vi "Complex Dot Product (no conjugate).vi"(2 "Y Vector":cdb[](array[numeric]), 3 "X Vector":cdb[](array[numeric])) -> (0 "error":i32, 1 "X * Y":cdb)   [LabVIEW 2018, in "NI_AALBase.lvlib"]
doc: "Computes the dot product of <B>X Vector</B> and <B>Y Vector</B>. You can use this polymorphic VI to compute a real dot product or a complex dot product. The data types you wire to the <B>X Vector</B> and <B>Y Vector</B> inputs determine the polymorphic instance to use."
uses:
  NI_AALBase.lvlib
  <resource>/lvanlys.dll
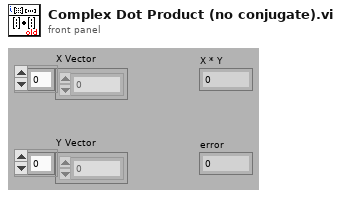
[diagram p1: front panel]
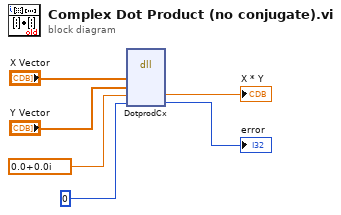
[diagram p0: block diagram]
diagram:
  n1 = dll-call lib="C:/Program Files (x86)/National Instruments/LabVIEW 2018/resource/lvanlys.*" fn="DotprodCx"("X Vector"="X Vector", "Y Vector"="Y Vector", cdb 0.0+0.0i, 0) -> (→"X * Y":cdb, →"error":i32)  [unwired: 6 in, 2 out]
